vi "ex3.1.vi"() -> ()   [LabVIEW 2015]
uses:
  <vilib>/eio/EIONode/EIONode.xnode
  <vilib>/rvi/eio/common/nirviEmuTemplateMethod_errors.vi
panel:
  out "Waveform Chart":i16(graph)
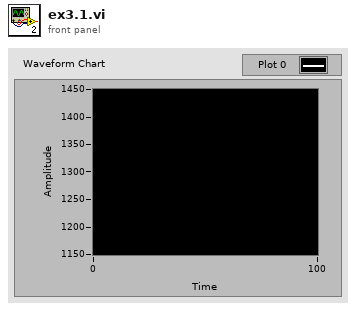
[diagram p1: front panel]
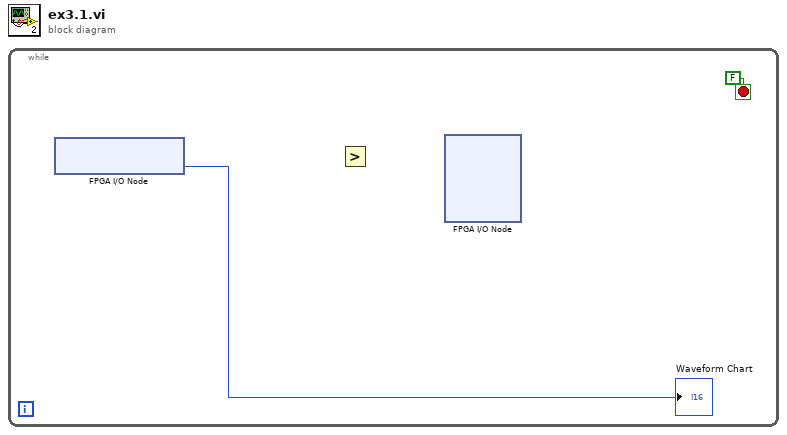
[diagram p0: block diagram]
diagram:
  n1 = while {
    stop <- FALSE ("Boolean") stop-if-true
    n2 = xnode "FPGA I/O Node"() -> ("ConnectorC/AI0"=→"Waveform Chart":i16)  [unwired: 1 in, 1 out]
    n3 = Greater?() -> ()  [unwired: 2 in, 1 out]
    n4 = xnode "FPGA I/O Node"() -> ()  [unwired: 8 in, 4 out]
  }
